vi "SetXL_CellValues_2D_String.vi"(6 "data":string[][](array[string]), 8 "error in":errorcluster, 9 "End":cluster{"Column":i32, "Row":i32}, 10 "Start":cluster{"Column":i32, "Row":i32}, 11 "Refnum Cluster In":T1) -> (0 "error out":errorcluster, 3 "Refnum Cluster Out":T1)   [LabVIEW 2015]
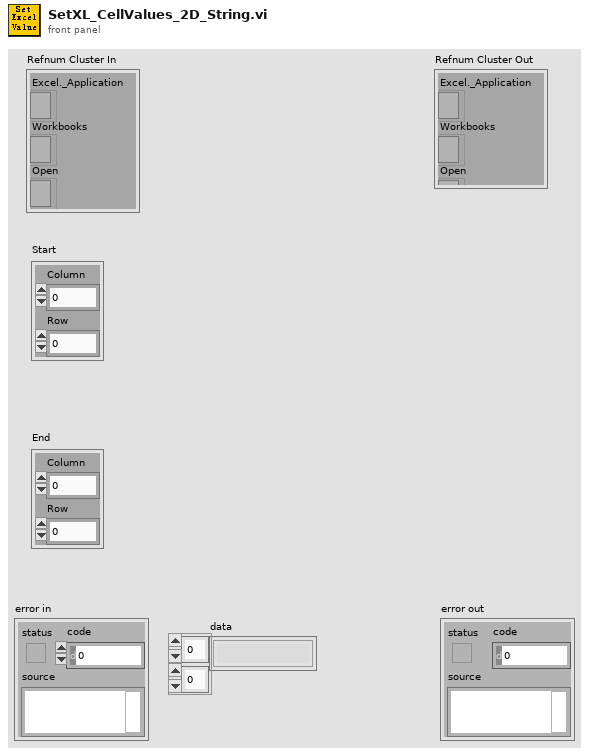
[diagram p1: front panel]
types:
  T1 = cluster{"Excel._Application":refnum<k7>, "Workbooks":refnum<k7>, "Open":refnum<k7>, "Worksheets":refnum<k7>, "Excel._Worksheet":refnum<k7>}
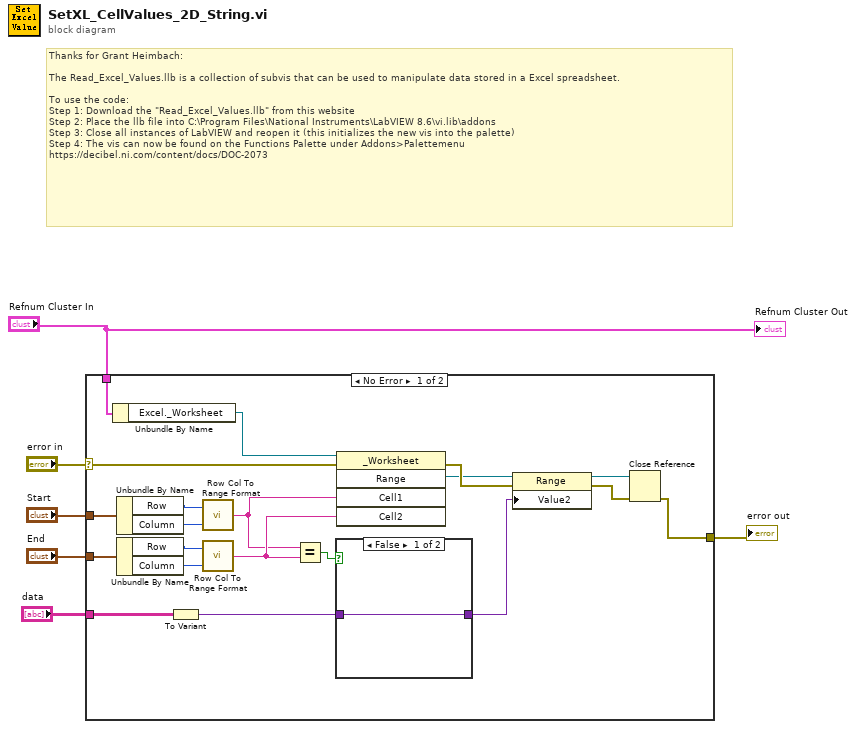
[diagram p0: block diagram]
diagram:
  # "Thanks for Grant Heimbach: \n\nThe Read_Excel_Values.llb is a collection of subvis that can be used to manipulate data stored in a Excel spreadsheet.\n \nTo use the code:\nStep 1: Download the \"Read_Excel_Values.llb\" from this website\nStep 2: Place the llb file into C:\\Program Files\\National Instruments\\LabVIEW 8.6\\vi.lib\\addons\nStep 3: Close all instances of LabVIEW and reopen it (this initializes the new vis into the palette)\nStep 4: The vis can now be found on the Functions Palette under Addons>Palettemenu\nhttps://decibel.ni.com/content/docs/DOC-2073"
  n1 = case shown="No Error" "error in" {
    selector: "error in" -> [w26 w29]
    tunnel: "Start" -> [w21 _]
    tunnel: "End" -> [w18 _]
    tunnel: [w7 w29] -> w3
    tunnel: "Refnum Cluster In" -> [w13 _]
    tunnel: "data" -> [w11 _]
    frame No Error {
      n2 = Unbundle By Name(w13) -> ("Excel._Worksheet"=w12:refnum<k7>)
      n3 = Unbundle By Name(w21) -> ("Row"=w20:i32, "Column"=w19:i32)
      n4 = Unbundle By Name(w18) -> ("Row"=w17:i32, "Column"=w16:i32)
      n5 = To Variant(anything=w11) -> (Variant=w9:variant)
      n6 = call "Row Col To Range Format.vi"("Column"=w19, "Row"=w20) -> ("Output String"=w14:string)
      n7 = call "Row Col To Range Format.vi"("Column"=w16, "Row"=w17) -> ("Output String"=w15:string)
      n8 = Equal?(x=w14, y=w15) -> (x = y?=w10:bool)
      n9 = case shown="False" w10 {
        tunnel: w9 -> [w27 w28]
        tunnel: [w27 w28] -> w8
        frame False {
        }
        frame True {
        }
      }
      n10 = invoke class="_Worksheet" method="Range"(reference=w12, error in=w26, "Cell1"=w14, "Cell2"=w15) -> (error out=w25:errorcluster, "Range"=w24:refnum<k7>)  [unwired: 1 in, 3 out]
      n11 = property class="Range"(reference=w24, error in=w25, "Value2"=w8) -> (reference out=w23:refnum<k7>, error out=w22:errorcluster)
      n12 = Close Reference(reference=w23, error in (no error)=w22) -> (error out=w7:errorcluster)
    }
    frame Error {
    }
  }
  "error out" <- w3
  "Refnum Cluster Out" <- "Refnum Cluster In"
